vi "指令解析.vi"(7 "指令类型":enum16{"standard", "short", "long", "OSD"}(ring), 10 "参数字符串":string, 11 "指令数组输入":string[](array[string])) -> (3 "指令输出":string[](array[string]))   [LabVIEW 2016]
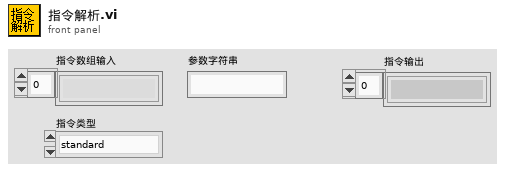
[diagram p1: front panel]
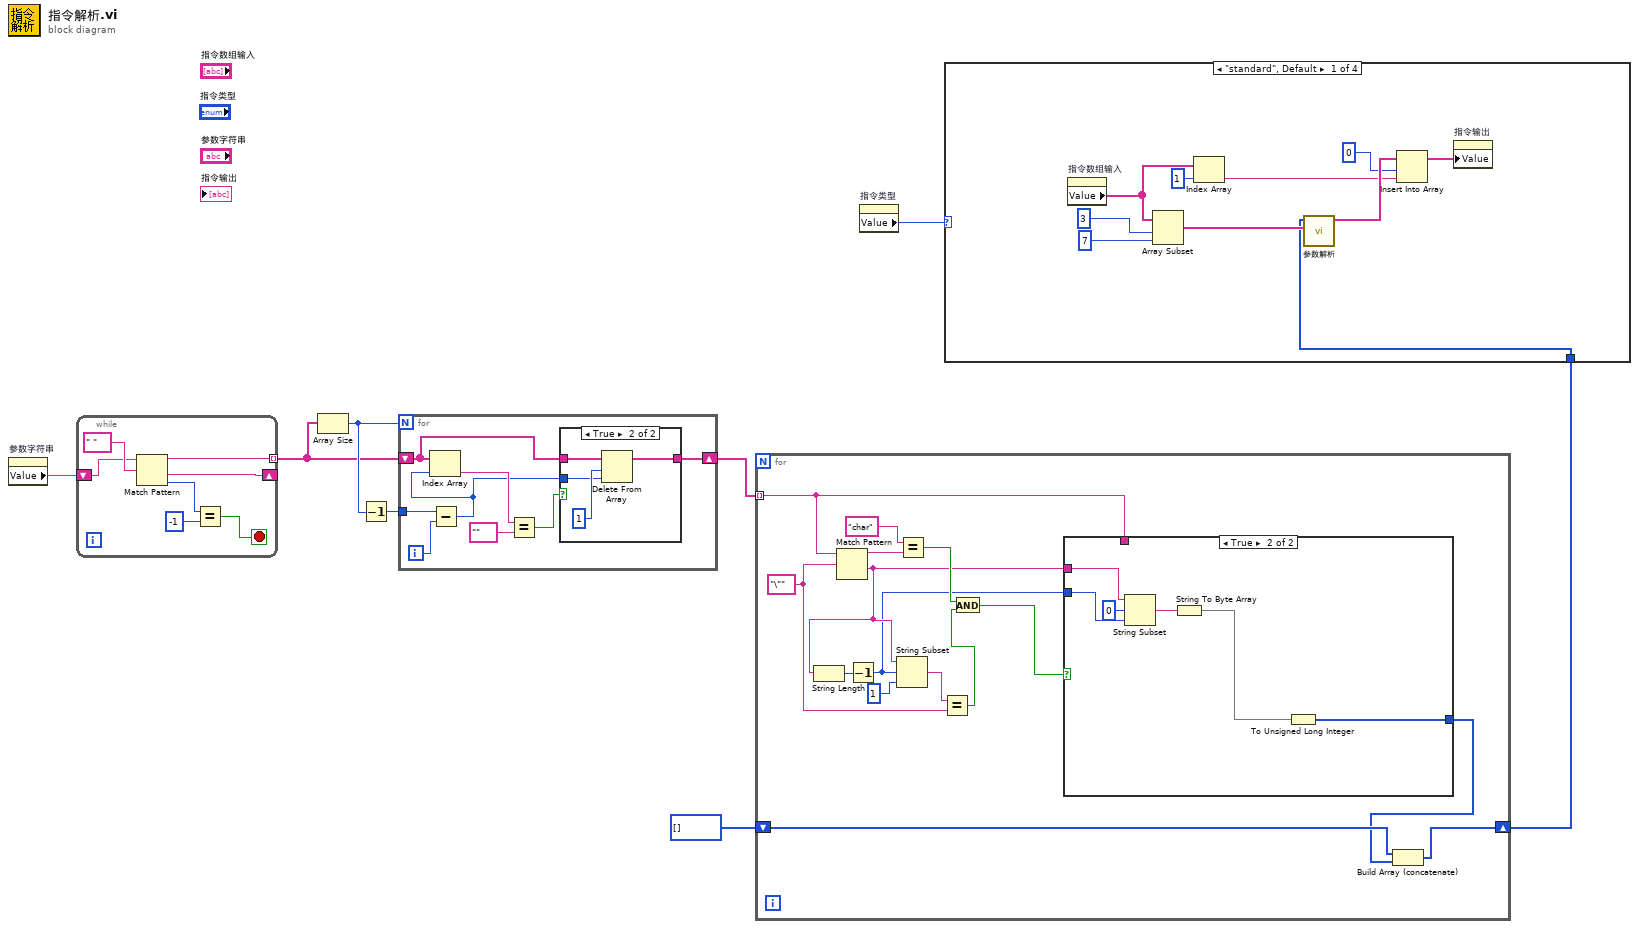
[diagram p0: block diagram]
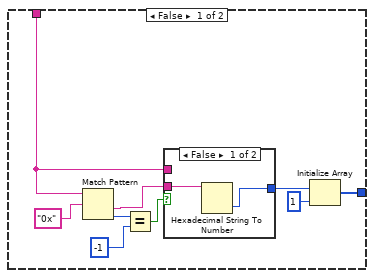
[diagram p2: hidden frame]
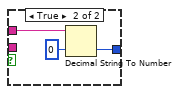
[diagram p3: hidden frame]
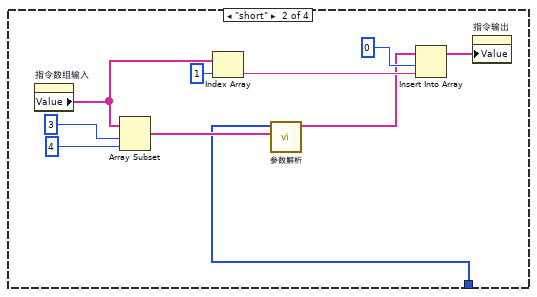
[diagram p5: hidden frame]
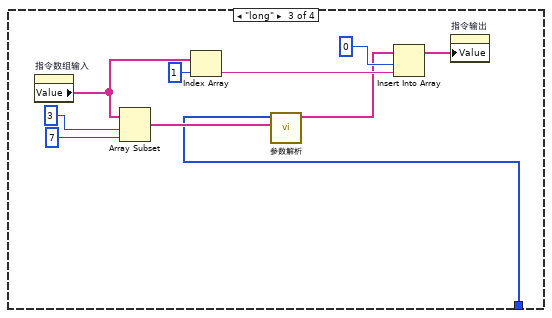
[diagram p6: hidden frame]
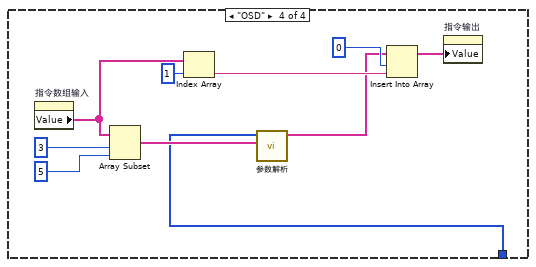
[diagram p7: hidden frame]
diagram:
  n1 = property on="参数字符串" class="Str"() -> ("Value"=w6:string)  [unwired: 2 in, 2 out]
  n2 = while {
    tunnel: [w11] -> w3 mode=indexing
    shift-right: [w10] -> _
    shift-left: w6 -> [w9]
    stop <- w12 stop-if-true
    n3 = Match Pattern(string=w9, regular expression=" " ("正则表达式")) -> (before substring=w11:string, after substring=w10:string, offset past match=w14:i32)  [unwired: 1 in, 1 out]
    n4 = Equal?(x=w14, y=-1) -> (x = y?=w12:bool)
  }
  n5 = Array Size(array=w3) -> (size(s)=w4:i32)
  n6 = Decrement(x=w4) -> (x-1=w5:i32)
  n7 = for {
    N: w4 -> [_]
    shift-right: [w17] -> w7
    shift-left: w3 -> [w18]
    tunnel: w5 -> [w21]
    i -> [w22]
    n8 = Subtract(x=w21, y=w22) -> (x-y=w16:i32)
    n9 = Index Array(array=w18, index=w16) -> (element=w20:string)
    n10 = Equal?(x=w20, y="") -> (x = y?=w19:bool)
    n11 = case shown="True" w19 {
      tunnel: w18 -> [w24 w28]
      tunnel: [w24 w27] -> w17
      tunnel: w16 -> [_ w25]
      frame False {
      }
      frame True {
        n12 = Delete From Array(array=w28, length=1 ("长度"), index=w25) -> (array with subset deleted=w27:string[])  [unwired: 1 out]
      }
    }
  }
  n13 = for {
    tunnel: w7 -> [w43] mode=indexing
    shift-right: [w30] -> w1
    shift-left: u32[] [] -> [w31]
    w39 = "\"" ("regular expression")
    n14 = Match Pattern(string=w43, regular expression=w39) -> (before substring=w37:string, after substring=w33:string)  [unwired: 1 in, 2 out]
    n15 = String Length(string=w33) -> (length=w42:i32)
    n16 = Decrement(x=w42) -> (x-1=w32:i32)
    n17 = String Subset(string=w33, offset (0)=w32, length (rest)=1 ("length (rest)")) -> (substring=w40:string)
    n18 = Equal?(x="char", y=w37) -> (x = y?=w36:bool)
    n19 = Equal?(x=w40, y=w39) -> (x = y?=w35:bool)
    n20 = And(x=w36, y=w35) -> (x .and. y?=w34:bool)
    n21 = case shown="True" w34 {
      tunnel: [w45 w58] -> w29
      tunnel: w43 -> [w47 _]
      tunnel: w33 -> [_ w63]
      tunnel: w32 -> [_ w62]
      frame False {
        n22 = Match Pattern(string=w47, regular expression="0x" ("正则表达式")) -> (after substring=w49:string, offset past match=w52:i32)  [unwired: 1 in, 2 out]
        n23 = Equal?(x=w52, y=-1) -> (x = y?=w51:bool)
        n24 = case shown="False" w51 {
          tunnel: w47 -> [_ w57]
          tunnel: [w54 w56] -> w46
          tunnel: w49 -> [w53 _]
          frame False {
            n25 = Hexadecimal String To Number(string=w53) -> (number=w54:u32)  [unwired: 2 in, 1 out]
          }
          frame True {
            n26 = Decimal String To Number(string=w57, default (0L)=u32 0 ("默认(0 I32)")) -> (number=w56:u32)  [unwired: 1 in, 1 out]
          }
        }
        n27 = Initialize Array(w46, 1 ("dimension size")) -> (w45:u32[])
      }
      frame True {
        n28 = String Subset(string=w63, offset (0)=0, length (rest)=w62) -> (substring=w60:string)
        n29 = String To Byte Array(string=w60) -> (unsigned byte array=w59:u8[])
        n30 = To Unsigned Long Integer(number=w59) -> (unsigned 32bit integer=w58:u32[])
      }
    }
    n31 = Build Array (concatenate)(w31, w29) -> (w30:u32[])
  }
  n32 = property on="指令类型" class="Enum (strict)"() -> ("Value"=w8:enum16{"standard", "short", "long", "OSD"})  [unwired: 2 in, 2 out]
  n33 = case shown="\"standard\", Default" w8 {
    tunnel: w1 -> [w64 w74 w84 w94]
    frame "standard", Default {
      n34 = property on="指令数组输入" class="Arr (strict)"() -> ("Value"=w70:string[])  [unwired: 2 in, 2 out]
      n35 = Array Subset(array=w70, index=3 ("索引"), length=7 ("长度")) -> (w72:string[])
      n36 = Index Array(array=w70, index=1) -> (element=w67:string)
      n37 = call "参数解析.vi"("指令格式"=w72, "参数数组"=w64) -> ("解析指令数组"=w68:string[])  [unwired: 9 in]
      n38 = Insert Into Array(array=w68, index=0, new element=w67) -> (w65:string[])
      n39 = property on="指令输出" class="Arr (strict)"("Value"=w65) -> ()  [unwired: 2 in, 2 out]
    }
    frame "short" {
      n40 = property on="指令数组输入" class="Arr (strict)"() -> ("Value"=w76:string[])  [unwired: 2 in, 2 out]
      n41 = Array Subset(array=w76, index=3 ("索引"), length=4 ("长度")) -> (w82:string[])
      n42 = Index Array(array=w76, index=1) -> (element=w79:string)
      n43 = call "参数解析.vi"("指令格式"=w82, "参数数组"=w74) -> ("解析指令数组"=w75:string[])  [unwired: 9 in]
      n44 = Insert Into Array(array=w75, index=0, new element=w79) -> (w77:string[])
      n45 = property on="指令输出" class="Arr (strict)"("Value"=w77) -> ()  [unwired: 2 in, 2 out]
    }
    frame "long" {
      n46 = property on="指令数组输入" class="Arr (strict)"() -> ("Value"=w86:string[])  [unwired: 2 in, 2 out]
      n47 = Array Subset(array=w86, index=3 ("索引"), length=7 ("长度")) -> (w93:string[])
      n48 = Index Array(array=w86, index=1) -> (element=w89:string)
      n49 = call "参数解析.vi"("指令格式"=w93, "参数数组"=w84) -> ("解析指令数组"=w85:string[])  [unwired: 9 in]
      n50 = Insert Into Array(array=w85, index=0, new element=w89) -> (w87:string[])
      n51 = property on="指令输出" class="Arr (strict)"("Value"=w87) -> ()  [unwired: 2 in, 2 out]
    }
    frame "OSD" {
      n52 = property on="指令数组输入" class="Arr (strict)"() -> ("Value"=w96:string[])  [unwired: 2 in, 2 out]
      n53 = Array Subset(array=w96, index=3 ("索引"), length=5 ("长度")) -> (w103:string[])
      n54 = Index Array(array=w96, index=1) -> (element=w100:string)
      n55 = call "参数解析.vi"("指令格式"=w103, "参数数组"=w94) -> ("解析指令数组"=w95:string[])  [unwired: 9 in]
      n56 = Insert Into Array(array=w95, index=0, new element=w100) -> (w99:string[])
      n57 = property on="指令输出" class="Arr (strict)"("Value"=w99) -> ()  [unwired: 2 in, 2 out]
    }
  }
